vi "One Ball.vi"   [LabVIEW 2013]
uses:
  Robot Global Data.vi
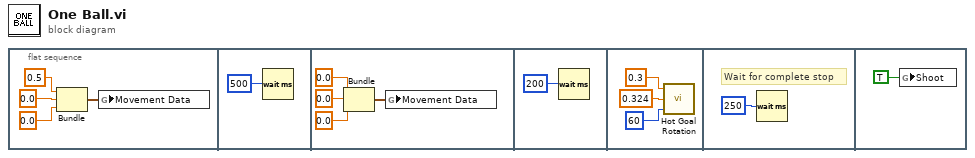
[diagram p0: block diagram]
diagram:
  n1 = flat-sequence {
    frame #0 {
      n2 = Bundle(0.5, 0.0, 0.0) -> (w4:cluster{dbl, dbl, dbl})  [unwired: 1 in]
      n3 = global write "Robot Global Data.vi" "Movement Data"(w4) -> ()
    }
    frame #1 {
      n4 = Wait (ms)(milliseconds to wait=u32 500) -> ()  [unwired: 1 out]
    }
    frame #2 {
      n5 = Bundle(0.0, 0.0, 0.0) -> (w9:cluster{dbl, dbl, dbl})  [unwired: 1 in]
      n6 = global write "Robot Global Data.vi" "Movement Data"(w9) -> ()
    }
    frame #3 {
      n7 = Wait (ms)(milliseconds to wait=u32 200) -> ()  [unwired: 1 out]
    }
    frame #4 {
      n8 = call "Hot Goal Rotation.vi"("Gyro Refresh Rate (Hz)"=u32 60, "Degrees to rotate"=0.324, "Rotate Power"=0.3) -> ()
    }
    frame #5 {
      # "Wait for complete stop"
      n9 = Wait (ms)(milliseconds to wait=u32 250) -> ()  [unwired: 1 out]
    }
    frame #6 {
      n10 = global write "Robot Global Data.vi" "Shoot"(TRUE ("Shoot")) -> ()
    }
  }
